vi "circle scan.vi"(9 "x-y phase shift (*2^16/2*pi)":u16=16384, 10 "tracking settings":T1={"scan radius"=0, "2^16/lines per revolution"=1394, "gx"=0.0, "rtw"=0.0, "lines per revolution"=47, "vel diff"=0.0, "Dx - for pos only k-f"=0.0}, 11 "new line":bool) -> (1 "line counter":u8, 2 "y value":i16, 3 "x value":i16)   [LabVIEW 2010]
uses:
  polar tracking settings.ctl
  <vilib>/rvi/FXPMathLib/FxpInterpret/XNode/nifxpmath_Interpret.xnode
  <vilib>/rvi/FXPMathLib/FxpMul/XNode/nifxpmath_Multiplier.xnode
  <vilib>/rvi/FXPMathLib/FxpMul/subVIs/nifxpmath_Mul_SimConfig.ctl
  <vilib>/fxp/LVFixedPointQuantizationPolicyTypeDef.ctl
  <vilib>/fxp/LVFixedPointOverflowPolicyTypeDef.ctl
  <vilib>/rvi/FXPMathLib/FxpMul/simVIs/DllFxpMulTemp_sub.vi
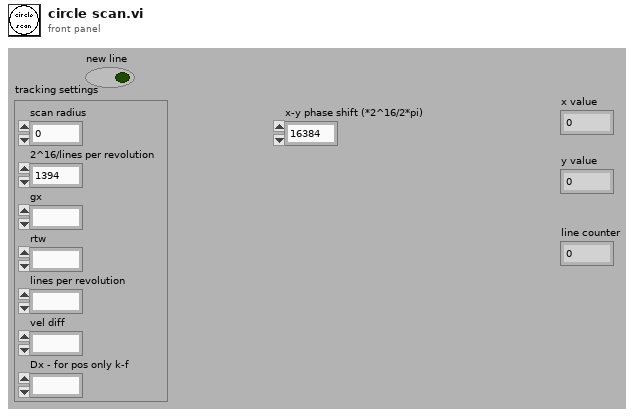
[diagram p1: front panel]
types:
  T1 = typedef "polar tracking settings.ctl" = cluster{"scan radius":u16, "2^16/lines per revolution":u16, "gx":fxp<+,16,8>, "rtw":fxp<+,16,26>, "lines per revolution":u8, "vel diff":fxp<+,24,-22>, "Dx - for pos only k-f":fxp<+,32,19>}
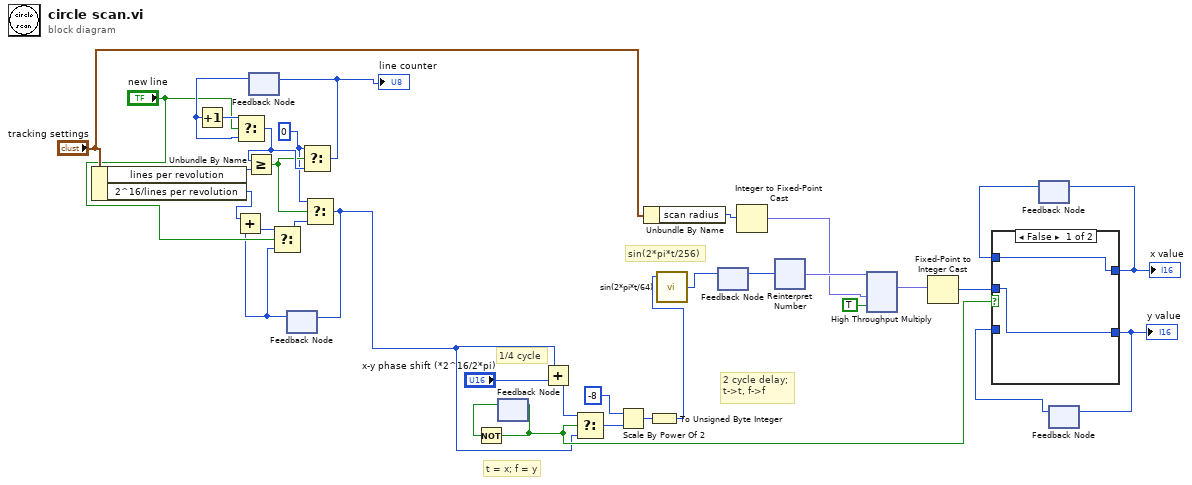
[diagram p0: block diagram]
diagram:
  w13 = u8 0 ("t")
  # "sin(2*pi*t/256)"
  # "2 cycle delay;\nt->t, f->f"
  # "t = x; f = y"
  # "1/4 cycle"
  n1 = Unbundle By Name("tracking settings") -> ("lines per revolution"=w19:u8, "2^16/lines per revolution"=w12:u16)
  n2 = feedback #1() -> (w17:u8)  [unwired: 1 in]
  n3 = Increment(x=w17) -> (x+1=w18:u8)
  n4 = Select(t=w18, s="new line", f=w17) -> (s? t:f=w16:u8)
  n5 = Greater Or Equal?(x=w16, y=w19) -> (x >= y?=w14:bool)
  n6 = feedback #2() -> (w4:u16)  [unwired: 1 in]
  n7 = Add(x=w12, y=w4) -> (x+y=w5:u16)
  n8 = Select(t=w5, s="new line", f=w4) -> (s? t:f=w3:u16)
  n9 = Select(t=w13, s=w14, f=w16) -> (s? t:f=w15:u8)
  "line counter" <- w15
  n10 = feedback-in #1(w15) -> ()
  n11 = Select(t=w13, s=w14, f=w3) -> (s? t:f=w9:u16)
  n12 = feedback-in #2(w9) -> ()
  n13 = feedback #3() -> (w32:bool)  [unwired: 1 in]
  n14 = Not(x=w32) -> (.not. x?=w25:bool)
  n15 = feedback-in #3(w25) -> ()
  n16 = Add(x=w9, y="x-y phase shift (*2^16/2*pi)") -> (x+y=w31:u16)
  n17 = Select(t=w31, s=w25, f=w9) -> (s? t:f=w2:u16)
  n18 = Scale By Power Of 2(n=-8, x=w2) -> (x*2^n=w8:u16)
  n19 = Unbundle By Name("tracking settings") -> ("scan radius"=w10:u16)
  n20 = To Unsigned Byte Integer(number=w8) -> (unsigned 8bit integer=w1:u8)
  n21 = call "sin(2*pi*t/64)"("address"=w1) -> ("data out"=w34:i8)  [unwired: 8 in]
  n22 = feedback-in #4(w34) -> ()
  n23 = feedback #4() -> (w33:i8)  [unwired: 1 in]
  n24 = Integer to Fixed-Point Cast(integer=w10) -> (fixed-point=w28:fxp<+,16,16>)  [unwired: 1 in]
  n25 = xnode "Reinterpret Number"("x"=w33) -> ("y"=w29:fxp<+/-,8,1>)
  n26 = xnode "High Throughput Multiply"("x"=w29, "y"=w28, "input valid"=TRUE) -> ("x*y"=w26:fxp<+/-,16,16>)  [unwired: 1 in, 2 out]
  n27 = Fixed-Point to Integer Cast(1:w26) -> (0:w24:i16)
  n28 = feedback #5() -> (w22:i16)  [unwired: 1 in]
  n29 = feedback #6() -> (w20:i16)  [unwired: 1 in]
  n30 = case shown="False" w25 {
    tunnel: w24 -> [w36 w38]
    tunnel: [w35 w38] -> w23
    tunnel: [w36 w37] -> w21
    tunnel: w22 -> [w35 _]
    tunnel: w20 -> [_ w37]
    frame False {
    }
    frame True {
    }
  }
  "x value" <- w23
  "y value" <- w21
  n31 = feedback-in #5(w23) -> ()
  n32 = feedback-in #6(w21) -> ()
